vi "Connect I2C Slave.vi"(8 "error in (no error)":errorcluster, 10 "I2C Slave Configuration":T1={"Address"=56, "Clock Rate (kHz)"=100, "Address Size"=0} {"Address Size" items=["7 Bits", "10 Bits"]; "Address" format="%.0x"}) -> (0 "error out":errorcluster, 2 "i2c configuration":T2)   [LabVIEW 2016]
uses:
  <vilib>/ni845x/ni845x.llb/ni845xI2cConfiguration.ctl
  Type Definitions/I2C Slave Configuration.ctl
  <resource>/objmgr/NI845x.rc
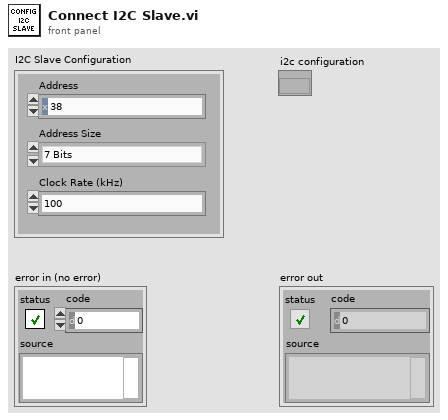
[diagram p1: front panel]
types:
  T1 = typedef "I2C Slave Configuration.ctl" = cluster{"Address":u16, "Clock Rate (kHz)":u16, "Address Size":i32}
  T2 = typedef "ni845xI2cConfiguration.ctl" = refnum<k20>
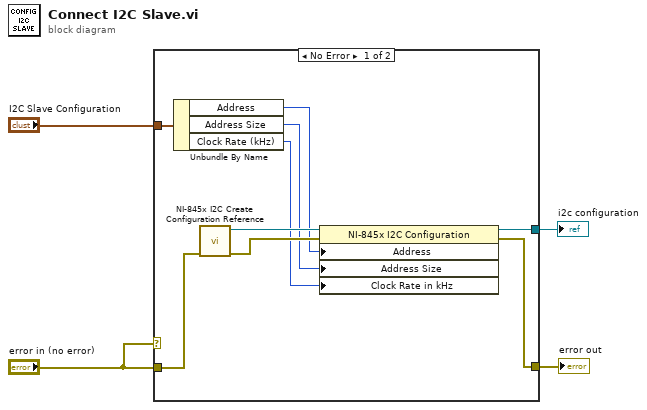
[diagram p0: block diagram]
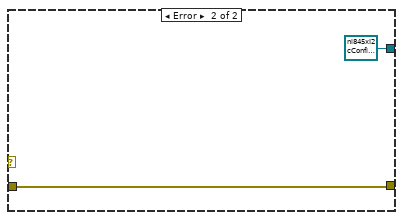
[diagram p2: hidden frame]
diagram:
  n1 = case shown="No Error" "error in (no error)" {
    tunnel: [w13 w15] -> w4
    tunnel: [w12 T2 refnum ("i2c configuration")] -> w3
    tunnel: "error in (no error)" -> [w9 w15]
    tunnel: "I2C Slave Configuration" -> [w8 _]
    frame No Error {
      n2 = Unbundle By Name(w8) -> ("Address"=w7:u16, "Address Size"=w6:i32, "Clock Rate (kHz)"=w5:u16)
      n3 = call <vilib>:"NI-845x I2C Create Configuration Reference.vi"("error in (no error)"=w9) -> ("error out"=w11:errorcluster, "i2c configuration"=w10:T2)  [unwired: 9 out]
      n4 = property on="Property Node" class="NI-845x I2C Configuration"(reference=w10, error in=w11, "Address"=w7, "Address Size"=w6, "Clock Rate in kHz"=w5) -> (reference out=w12:T2, error out=w13:errorcluster)
    }
    frame Error {
    }
  }
  "error out" <- w4
  "i2c configuration" <- w3
